vi "AuMT8852B Carrier Drift Results Query.vi"(8 "error in (no error)":errorcluster, 11 "VISA session":refnum<visa-resource-name>) -> (0 "error out":errorcluster, 2 "error code":i32, 3 "VISA session out":refnum<visa-resource-name>, 4 "Results":T1 {"Drift rate (KHz)" format="%.2f"; "Five slot packet drift (KHz)" format="%.2f"; "Three slot packet drift (KHz)" format="%.2f"; "One slot packet drift (KHz)" format="%.2f"})   [LabVIEW 2017]
doc: "Anritsu MT8852B Bluetooth Tester\n\nReturns the results of the Carrier Drift test.\n\nOUTPUTS\nResults - measurements made during the test."
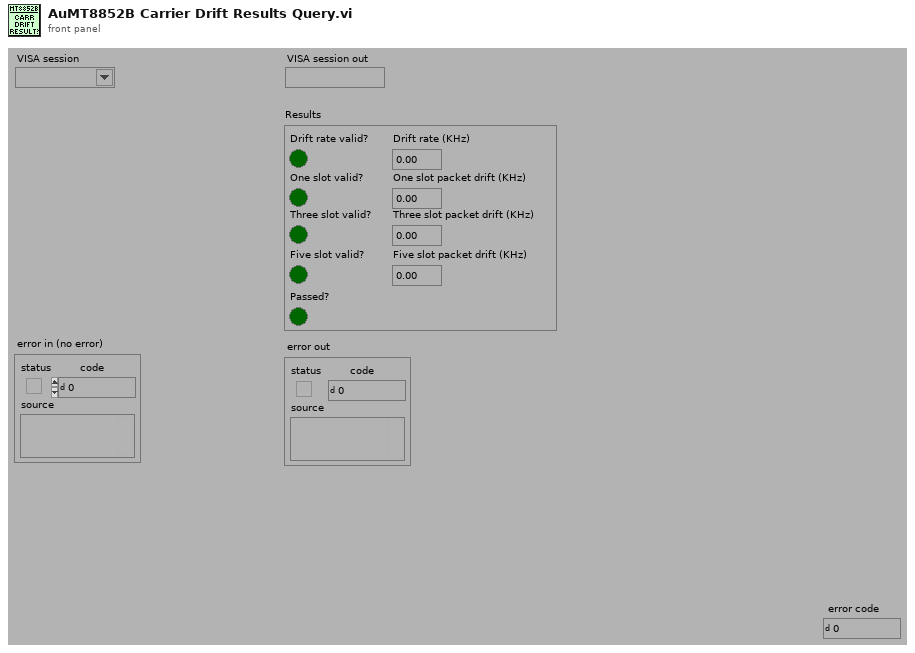
[diagram p1: front panel]
types:
  T1 = cluster{"Passed?":bool, "Five slot valid?":bool, "Three slot valid?":bool, "One slot valid?":bool, "One slot packet drift (KHz)":dbl, "Three slot packet drift (KHz)":dbl, "Five slot packet drift (KHz)":dbl, "Drift rate valid?":bool, "Drift rate (KHz)":dbl}
  T2 = enum16{"Simulate", "Range check", "Cache", "Query instrument status"}
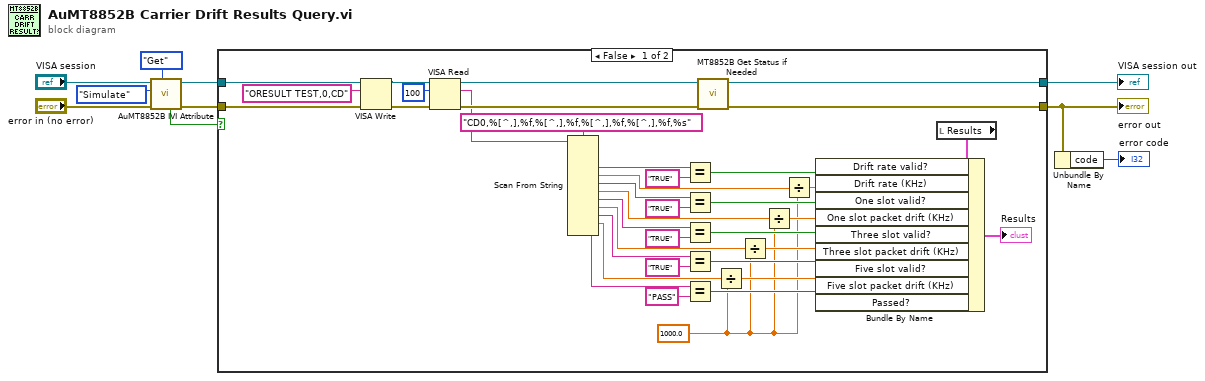
[diagram p0: block diagram]
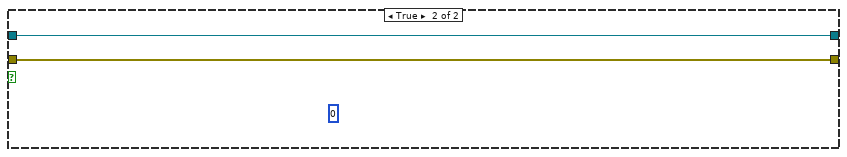
[diagram p2: hidden frame]
diagram:
  n1 = call <instrlib>:"AuMT8852B IVI Attribute.vi"("Set/Get (Set)"=enum16{"Set", "Get"}."Get", "error in (no error)"="error in (no error)", "Flag (Simulate)"=T2."Simulate", "VISA session"="VISA session") -> ("error out"=w7:errorcluster, "VISA session out"=w9:refnum<visa-resource-name>, "Value out"=w3:bool)  [unwired: 5 in]
  n2 = case shown="False" w3 {
    tunnel: [w39 w50] -> w10
    tunnel: [w38 w49] -> w1
    tunnel: w9 -> [w47 w50]
    tunnel: w7 -> [w46 w49]
    frame False {
      w11 = 1000.0 ("y")
      n3 = VISA Write(VISA resource name=w47, write buffer="ORESULT TEST,0,CD" ("write buffer (\"\")"), error in (no error)=w46) -> (VISA resource name out=w45:refnum<visa-resource-name>, error out=w44:errorcluster)  [unwired: 1 out]
      n4 = VISA Read(VISA resource name=w45, byte count=u32 100 ("byte count (0)"), error in (no error)=w44) -> (VISA resource name out=w25:refnum<visa-resource-name>, read buffer=w23:string, error out=w24:errorcluster)  [unwired: 1 out]
      n5 = Scan From String(format string="CD0,%[^,],%f,%[^,],%f,%[^,],%f,%[^,],%f,%s" ("Format String"), input string=w23) -> (output 1=w21:string, output 2=w18:dbl, output 3=w33:string, output 4=w16:dbl, output 5=w36:string, output 6=w15:dbl, output 7=w28:string, output 8=w12:dbl, output 9=w35:string)  [unwired: 11 in, 3 out]
      n6 = Equal?(x=w21, y="TRUE") -> (x = y?=w20:bool)
      n7 = Equal?(x=w33, y="TRUE") -> (x = y?=w32:bool)
      n8 = Equal?(x=w36, y="TRUE") -> (x = y?=w31:bool)
      n9 = Equal?(x=w28, y="TRUE") -> (x = y?=w29:bool)
      n10 = Equal?(x=w35, y="PASS") -> (x = y?=w34:bool)
      n11 = call <instrlib>:"MT8852B Get Status if Needed.vi"("error in (no error)"=w24, "VISA session"=w25) -> ("error out"=w38:errorcluster, "VISA session out"=w39:refnum<visa-resource-name>)  [unwired: 8 in]
      n12 = Divide(x=w12, y=w11) -> (x/y=w13:dbl)
      n13 = Divide(x=w15, y=w11) -> (x/y=w14:dbl)
      n14 = Divide(x=w16, y=w11) -> (x/y=w17:dbl)
      n15 = Divide(x=w18, y=w11) -> (x/y=w19:dbl)
      n16 = local read "Results"() -> (w41:T1)
      n17 = Bundle By Name(cluster=w41, "Drift rate valid?"=w20, "Drift rate (KHz)"=w19, "One slot valid?"=w32, "One slot packet drift (KHz)"=w17, "Three slot valid?"=w31, "Three slot packet drift (KHz)"=w14, "Five slot valid?"=w29, "Five slot packet drift (KHz)"=w13, "Passed?"=w34) -> (→"Results":T1)
    }
    frame True {
      (unwired) u8 0
    }
  }
  "error out" <- w1
  "VISA session out" <- w10
  n18 = Unbundle By Name(w1) -> ("code"=→"error code":i32)
